vi "SendEmail.vi"(8 "Error in (no error)":errorcluster, 10 "Array log in":T1[](array[typedef]) {"Priority" items=["EMERGENCY", "ALERT", "CRITICAL", "ERROR", "WARNING", "NOTICE", "INFO", "DEBUG"]}, 11 "LogWriterEmail in":refnum<class "LogWriterEmail.lvclass">) -> (0 "Error out":errorcluster, 3 "LogWriterEmail out":refnum<class "LogWriterEmail.lvclass">)   [LabVIEW 2011, in "LogWriterEmail.lvclass"]
uses:
  LogWriterEmail.lvclass
  Log/LogCluster.ctl
  Log/PrioritiesRing.ctl
  LogWriterEmail.lvclass/LogWriterEmail.ctl
  Formatter/LogFormatterInterface/LogFormatterInterface.lvclass
  <vilib>/Utility/SMTP/NI_SMTPEmail.lvlib
  LogWriterInterface/LogWriterInterface.lvclass
  Log/Log.lvclass
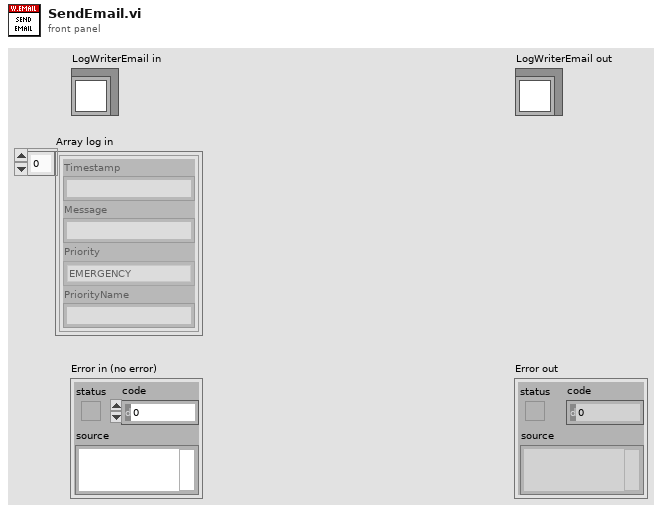
[diagram p1: front panel]
types:
  T1 = typedef "Log.lvclass/LogCluster.ctl" = cluster{"Timestamp":string, "Message":string, "Priority":T2, "PriorityName":string}
  T2 = typedef "Log.lvclass/PrioritiesRing.ctl" = u32
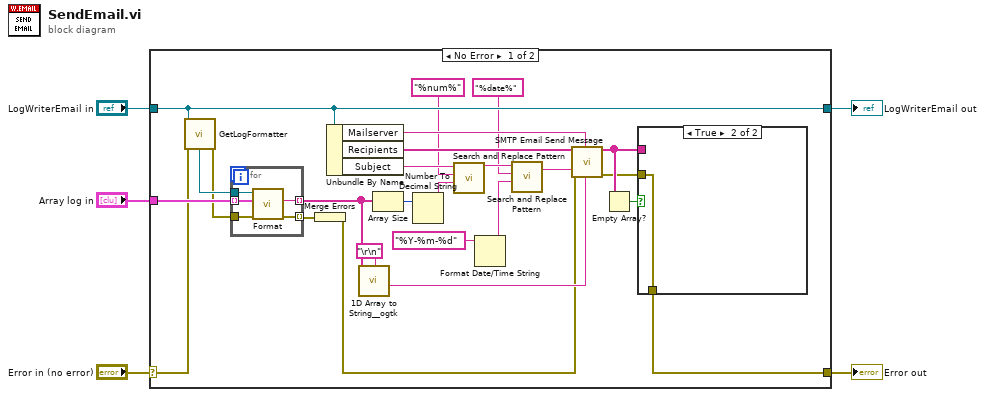
[diagram p0: block diagram]
diagram:
  n1 = case shown="No Error" "Error in (no error)" {
    selector: "Error in (no error)" -> [w26 w39]
    tunnel: [w16 w39] -> w4
    tunnel: [w27 w38] -> w2
    tunnel: "LogWriterEmail in" -> [w27 w38]
    tunnel: "Array log in" -> [w28 _]
    frame No Error {
      n2 = call "GetLogFormatter.vi"("Error in (no error)"=w26, "LogWriterInterface in"=w27) -> ("Error out"=w24:errorcluster, "LogFormatterInterface out"=w25:refnum<class "LogFormatterInterface.lvclass">)  [unwired: 7 in, 1 out]
      n3 = for {
        tunnel: w28 -> [w37] mode=indexing
        tunnel: [w36] -> w15 mode=indexing
        tunnel: w25 -> [w35]
        tunnel: w24 -> [w34]
        tunnel: [w33] -> w23 mode=indexing
        n4 = call-dynamic "Format.vi"("Error in (no error)"=w34, "Log in"=w37, "LogFormatterInterface in"=w35) -> ("Error out"=w33:errorcluster, "Log formatted"=w36:string)  [unwired: 6 in, 1 out]
      }
      n5 = Merge Errors(w23) -> (w20:errorcluster)
      n6 = Unbundle By Name(w27) -> ("Mailserver"=w30:string, "Recipients"=w29:string[], "Subject"=w14:string)
      n7 = call <userlib>:"1D Array to String__ogtk.vi"("delimiter (Tab)"="\r\n", "Array of Strings"=w15) -> ("delimited string"=w21:string)  [unwired: 9 in]
      n8 = Array Size(array=w15) -> (size(s)=w12:i32)
      n9 = Number To Decimal String(number=w12) -> (decimal integer string=w11:string)  [unwired: 1 in]
      n10 = call <vilib>:"Search and Replace Pattern.vi"("string"=w14, "regular expression (\"\")"="%num%" ("regular expression (\"\")"), "replace string (\"\")"=w11) -> ("result string"=w10:string)  [unwired: 2 in, 1 out]
      n11 = Format Date/Time String(time format string (%c)="%Y-%m-%d") -> (date/time string=w7:string)  [unwired: 2 in]
      n12 = call <vilib>:"Search and Replace Pattern.vi"("string"=w10, "regular expression (\"\")"="%date%" ("regular expression (\"\")"), "replace string (\"\")"=w7) -> ("result string"=w6:string)  [unwired: 2 in, 1 out]
      n13 = call <vilib>:"SMTP Email Send Message.vi"("recipients"=w29, "mail server"=w30, "subject ([No Subject])"=w6, "message"=w21, "error in (no error)"=w20) -> ("invalid recipients"=w18:string[], "error out"=w17:errorcluster)  [unwired: 9 in]
      n14 = Empty Array?(array=w18) -> (empty?=w19:bool)
      n15 = case shown="True" w19 {
        tunnel: w18 -> [_ _]
        tunnel: w17 -> [w31 w32]
        tunnel: [w31 w32] -> w16
        frame False {
          # "Error, email could\nnot be send to all \nrecipients"
        }
        frame True {
        }
      }
    }
    frame Error {
    }
  }
  "Error out" <- w4
  "LogWriterEmail out" <- w2
